vi "draw navigational matrix.vi"() -> ()   [LabVIEW 2009]
panel:
  out "miliseconds elapsed":u32
  in  "stop":bool
  in  "center":cluster{"x":i16, "y":i16}
  in  "angles":T1(array[cluster]) {"angle" scale=0.0..6.283184}
  out "Array":bool[][](array[boolean])
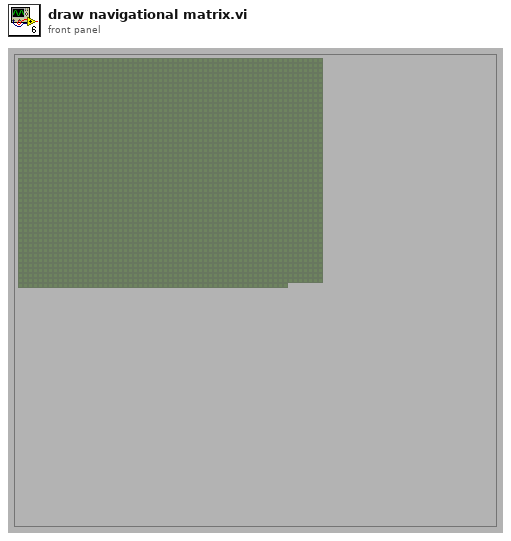
[diagram p1: front panel]
types:
  T1 = cluster{"spacing":i16, "radius":i16, "angle":dbl}[]
  T2 = cluster{"point":cluster{"x":i16, "y":i16}, "distance":u16, "theta":dbl}[]
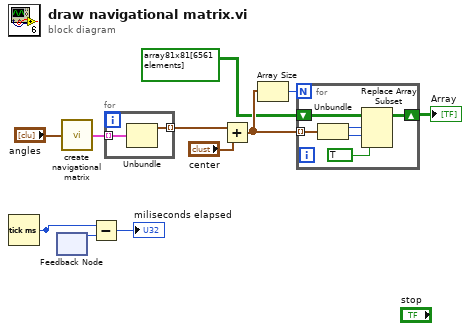
[diagram p0: block diagram]
diagram:
  n1 = Tick Count (ms)() -> (millisecond timer value=w3:u32)
  n2 = feedback #1() -> (w4:u32)  [unwired: 1 in]
  n3 = call "create navigational matrix.vi"("parameters"="angles") -> ("Array"=w8:T2)
  n4 = Subtract(x=w3, y=w4) -> (x-y=→"miliseconds elapsed":u32)
  n5 = for {
    tunnel: w8 -> [w13] mode=indexing
    tunnel: [w12] -> w7 mode=indexing
    n6 = Unbundle(w13) -> ("point"=w12:cluster{"x":i16, "y":i16})  [unwired: 2 out]
  }
  n7 = Add(x=w7, y="center") -> (x+y=w5:cluster{"x":i16, "y":i16}[])
  n8 = Array Size(array=w5) -> (size(s)=w6:i32)
  n9 = for {
    N: w6 -> [_]
    shift-right: [w17] -> w11
    shift-left: bool[][] array81x81[6561 elements] ("Array") -> [w19]
    tunnel: w5 -> [w16] mode=indexing
    n10 = Unbundle(w16) -> ("x"=w15:i16, "y"=w14:i16)
    n11 = Replace Array Subset(array=w19, new element=TRUE ("new element/subarray"), index (row)=w15, index (col)=w14) -> (w17:bool[][])
  }
  "Array" <- w11
